vi "HFRR ADV v012 new software.vi"() -> ()   [LabVIEW 2025] (continued)
              tunnel: w5189 -> [_ w5221]
              frame False {
              }
              frame True {
                n4036 = VISA Write(VISA resource name=w5225, write buffer=w5221, error in (no error)=w5224) -> (VISA resource name out=w5223:refnum<visa-resource-name>, error out=w5222:errorcluster)  [unwired: 1 out]
                n4037 = local write item#-1(FALSE ("WRITE")) -> ()
              }
            }
          }
          frame Error {
            w5313 = u16 10 items=["1.0"=10, "1.5"=15, "2.0"=20] ("stop bits (10: 1 bit)")
            n4038 = Wait (ms)(milliseconds to wait=u32 20) -> ()  [unwired: 1 out]
            n4039 = VISA Close(VISA resource name=w5315, error in (no error)=w5321) -> (error out=w5320:errorcluster)
            n4040 = call <vilib>:"Clear Errors.vi"("error in (no error)"=w5320) -> ("error out"=w5319:errorcluster)  [unwired: 5 in, 1 out]
            n4041 = call-poly "VISA Configure Serial Port"("timeout (10sec)"=u32 200, "Enable Termination\nChar (T)"=TRUE ("Enable Termination\nChar (T)"), "baud rate (9600)"=u32 921600, "error in (no error)"=w5319, "stop bits (10: 1 bit)"=w5313) -> ("VISA resource name"=w5311:refnum<visa-resource-name>, "VISA resource name out"=w5323:refnum<visa-resource-name>, "error out"=w5322:errorcluster)  [unwired: 8 in]
          }
        }
        n4042 = local read "Quit"() -> (w5163:bool)
      }
      n4043 = VISA Close(VISA resource name=w5158, error in (no error)=w5159) -> (error out=w5157:errorcluster)
      n4044 = call <vilib>:"Clear Errors.vi"("error in (no error)"=w5157) -> ()  [unwired: 5 in, 2 out]
    }
    frame Enabled {
    }
  }
  n4045 = disable-structure shown="Disabled" {
    disable-tunnel: _ -> [w5328 _]
    frame Disabled {
      n4046 = while {
        tunnel: [w5335] -> _
        shift-right: [w5332] -> w5325
        shift-left: _ -> [w5334]
        shift-right: [w5333] -> w5326
        shift-left: errorcluster {"status"=TRUE, "code"=0, "source"="Init"} ("error out") -> [w5331]
        tunnel: w5328 -> [_]
        i -> [w5335]
        stop <- w5329 stop-if-true
        n4047 = flat-sequence {
          tunnel: w5331 -> [w5426]
          tunnel: [w5426] -> w5330
          frame #0 {
            n4048 = Wait (ms)(milliseconds to wait=u32 50) -> ()  [unwired: 1 out]
          }
        }
        n4049 = case shown="No Error" w5330 {
          selector: w5330 -> [w5376 w5419]
          tunnel: w5334 -> [w5375 w5418]
          tunnel: [w5342 w5409] -> w5333
          tunnel: [w5343 w5417] -> w5332
          frame No Error {
            w5369 = T32 {"Mode"=enum."RTU", "Slave Address"=1} ("Serial Parameters")
            n4050 = call-poly <vilib>:"MB Serial Master Query (poly).vi"("VISA resource name"=w5375, "Starting Address"=i16 1000, "Quantity"=u16 1, "Timeout"=u32 1000, "error in"=w5376, "Serial Parameters"=w5369) -> ("VISA resource name out"=w5370:refnum<visa-resource-name>, "Input Registers"=w5372:u16[], "error out"=w5368:errorcluster)  [unwired: 10 in, 1 out]
            n4051 = Random Number (0-1)() -> (number: 0 to 1=w5357:dbl)
            n4052 = Index Array(array=w5372, index=0) -> (element=w5367:u16)
            n4053 = Subtract(x=w5357, y=0.5) -> (x-y=w5356:dbl)
            n4054 = Divide(x=w5367, y=10 ("index")) -> (x/y=w5361:dbl)
            n4055 = Multiply(x=w5356, y=0.5) -> (x*y=w5355:dbl)
            n4056 = Add(x=w5361, y=w5355) -> (x+y=w5360:dbl)
            n4057 = local read "Amb temp"() -> (w5344:dbl)
            n4058 = Multiply(x=w5360, y=0.2) -> (x*y=w5364:dbl)
            n4059 = Multiply(x=w5344, y=0.8) -> (x*y=w5362:dbl)
            n4060 = Add(x=w5364, y=w5362) -> (x+y=w5345:dbl)
            n4061 = local read "set temp old"() -> (w5339:dbl)
            n4062 = local write "Amb temp"(w5345) -> ()
            n4063 = Select(t="SetTemp 2", s="Heater", f=100.0) -> (s? t:f=w5340:dbl)
            n4064 = Not Equal?(x=w5340, y=w5339) -> (x != y?=w5338:bool)
            n4065 = case shown="True" w5338 {
              tunnel: w5370 -> [w5404 w5406]
              tunnel: [w5403 w5406] -> w5350
              tunnel: w5368 -> [w5402 w5405]
              tunnel: [w5401 w5405] -> w5348
              tunnel: w5340 -> [w5396 _]
              tunnel: w5369 -> [w5398 w5407]
              tunnel: [w5398 w5407] -> w5351
              frame True {
                n4066 = Multiply(x=w5396, y=10 ("index")) -> (x*y=w5395:dbl)
                n4067 = call-poly <vilib>:"MB Serial Master Query (poly).vi"("VISA resource name"=w5404, "Address"=u16 0, "Holding Register"=w5395, "Timeout"=u32 1000, "error in"=w5402, "Serial Parameters"=w5398) -> ("VISA resource name out"=w5403:refnum<visa-resource-name>, "error out"=w5401:errorcluster)  [unwired: 11 in, 1 out]
                "set temp old" <- w5396
              }
              frame False {
              }
            }
            n4068 = flat-sequence {
              tunnel: [w5377] -> _
              tunnel: [w5377] -> w5347
              tunnel: w5348 -> [w5377]
              frame #0 {
                n4069 = Wait (ms)(milliseconds to wait=u32 100) -> ()  [unwired: 1 out]
              }
            }
            n4070 = call "Elapsed Time12"("Time Target (s)"=2.0, "Auto Reset"=TRUE) -> ("Time has Elapsed"=w5352:bool)  [unwired: 10 in, 7 out]
            n4071 = case shown="True" w5352 {
              tunnel: w5351 -> [w5381 w5394]
              tunnel: [w5381 w5394] -> _
              tunnel: [w5380 w5392] -> w5343
              tunnel: w5350 -> [w5380 w5393]
              tunnel: [w5379 w5390] -> w5342
              tunnel: w5347 -> [w5379 w5391]
              frame False {
              }
              frame True {
                n4072 = call-poly <vilib>:"MB Serial Master Query (poly).vi"("VISA resource name"=w5393, "Starting Address"=i16 1003 ("Addr"), "Quantity"=u16 1, "Timeout"=u32 1000, "error in"=w5391, "Serial Parameters"=w5394) -> ("VISA resource name out"=w5392:refnum<visa-resource-name>, "Input Registers"=w5387:u16[], "error out"=w5390:errorcluster)  [unwired: 10 in, 1 out]
                n4073 = Index Array(array=w5387, index=0) -> (element=w5386:u16)
                n4074 = Divide(x=w5386, y=u16 10) -> (x/y=w5382:dbl)
                n4075 = local write "set temp old"(w5382) -> ()
                n4076 = local write "SetTemp"(w5382) -> ()
              }
            }
            "Error Code" <- w5342
            n4077 = Unbundle(w5342) -> ("status"=→"TK4 status":bool)  [unwired: 2 out]
            "SetTemp" <- "SetTemp 2"
          }
          frame Error {
            w5421 = u16 0 items=["None", "Odd", "Even", "Mark", "Space"] ("Parity")
            w5422 = u16 0 items=["None", "XON/XOFF", "RTS/CTS", "XON/XOFF & RTS/CTS", "DTR/DSR", "XON/XOFF & DTR/DSR"] ("Flow Control")
            n4078 = VISA Clear(VISA resource name=w5418, error in (no error)=w5419) -> (VISA resource name out=w5412:refnum<visa-resource-name>, error out=w5410:errorcluster)
            n4079 = VISA Close(VISA resource name=w5412, error in (no error)=w5410) -> (error out=w5411:errorcluster)
            n4080 = call <vilib>:"Clear Errors.vi"("error in (no error)"=w5411) -> ("error out"=w5420:errorcluster)  [unwired: 5 in, 1 out]
            n4081 = Unbundle By Name(T32 {"Mode"=enum."RTU", "Slave Address"=1} ("input cluster")) -> ("Mode"=w5423:enum16{"RTU", "ASCII"})
            n4082 = call <vilib>:"MB Serial Init.vi"("Timeout"=u32 100, "Flow Control"=w5422, "Mode"=w5423, "error in (no error)"=w5420, "Parity"=w5421, "Baud Rate"=u32 9600, "VISA resource name"="Lubrication System COM Port :") -> ("error out"=w5409:errorcluster, "VISA resource name out"=w5417:refnum<visa-resource-name>)  [unwired: 3 in]
            n4083 = local write "set temp old"(0.0 ("set temp old")) -> ()
            n4084 = Unbundle(w5409) -> ("status"=w5408:bool)  [unwired: 2 out]
            n4085 = case shown="True" w5408 {
              selector: w5408 -> [_ w5425]
              frame False {
              }
              frame True {
                n4086 = local write "TK4 status"(w5425) -> ()
              }
            }
          }
        }
        n4087 = local read "Quit"() -> (w5329:bool)
      }
      n4088 = VISA Close(VISA resource name=w5325, error in (no error)=w5326) -> (error out=w5324:errorcluster)
      n4089 = call <vilib>:"Clear Errors.vi"("error in (no error)"=w5324) -> ()  [unwired: 5 in, 2 out]
    }
    frame Enabled {
    }
  }
